vi "Explore Finite Precision Effects.vi"() -> ()   [LabVIEW 2023]
doc: "This example demonstrates the finite word length effects of fixed-point conversion by comparing the error signals of two fixed-point LMS adaptive filters. Each adaptive filter is identical except for the coefficients word length. The first filter has a coefficients word length of 24 bits, and the second filter has a coefficients word length of 16 bits.\n\nAfter you run this VI, this example displays the error signals of both filters. Notice that the error signal of the first filter is smaller than the error signal of the second filter. This difference shows how increasing the coefficients word length reduces errors during fixed-point processing. However, increasing the coefficients word length also increases the amount of hardware resources a filter requires.\n\nOn the block diagram of this example VI, double-click the AFT Simulate Fixed-Point FIR LMS Express VI to examine the settings of the fixed-point LMS adaptive filters. You also can modify the settings to find out how different settings affect the performance of the fixed-point adaptive filters."
uses:
  <vilib>/addons/Adaptive Filters/Utilities/AFT Fixed-Point Settings.ctl
  <vilib>/addons/Adaptive Filters/Utilities/AFT Algorithm.ctl
  <vilib>/addons/Adaptive Filters/Fixed-Point Simulation/LMS/AFT Simulate Fixed-Point FIR LMS.xnode
  <vilib>/addons/Adaptive Filters/NI_AdaptiveFilter.lvlib
  <vilib>/addons/Adaptive Filters/Utilities/AFT Simulation Info.ctl
panel:
  in  "Samples":i32=4096 min=100
  out "Error Signals":dbl[][](graph)
  # "Select Help>>Show Context Help and move the cursor over the VI icon of this example for more information."
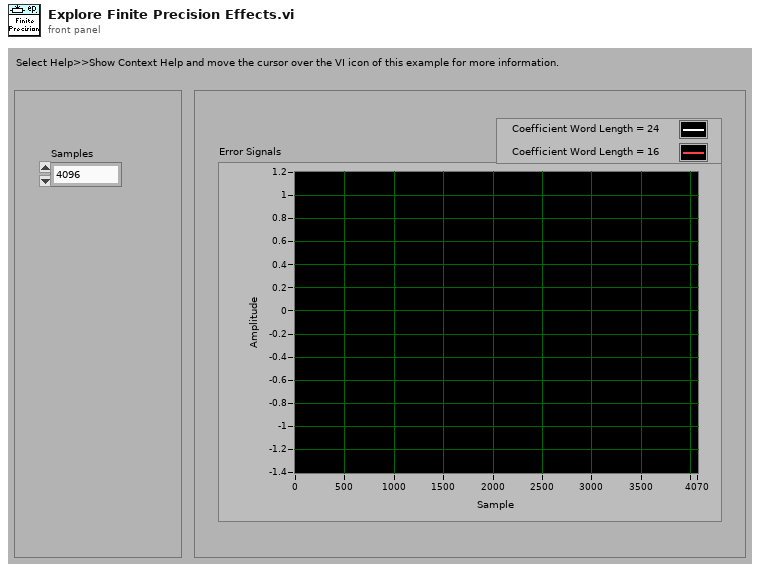
[diagram p1: front panel]
types:
  T1 = typedef "NI_AdaptiveFilter.lvlib/AFT Fixed-Point Settings.ctl" = cluster{"algorithm":u16, "filter length":i32, "step size":dbl, "encoding":cluster{"x(n) word length":i32, "x(n) integer word length":i32, "d(n) word length":i32, "d(n) integer word length":i32, "w(n) word length":i32, "w(n) integer word length":i32, "step size word length":i32, "step size integer word length":i32}}
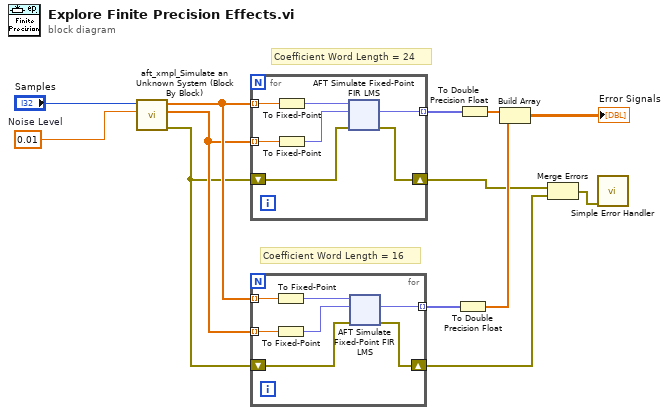
[diagram p0: block diagram]
diagram:
  w4 = 0.01  # Noise Level
  # "Coefficient Word Length = 16"
  # "Coefficient Word Length = 24"
  n1 = call "aft_xmpl_Simulate an Unknown System (Block By Block).vi"("noise level"=w4, "samples"="Samples") -> ("error out"=w1:errorcluster, "response signal"=w2:dbl[], "stimulus signal"=w3:dbl[])  [unwired: 2 in, 5 out]
  n2 = for {
    tunnel: w3 -> [w20] mode=indexing
    tunnel: w2 -> [w18] mode=indexing
    tunnel: [w16] -> w10 mode=indexing
    shift-right: [w15] -> w8
    shift-left: w1 -> [w14]
    n3 = To Fixed-Point(number=w20) -> (fixed-point=w19:fxp<+/-,24,4>)  [unwired: 1 out]
    n4 = To Fixed-Point(number=w18) -> (fixed-point=w17:fxp<+/-,24,4>)  [unwired: 1 out]
    n5 = xnode "AFT Simulate Fixed-Point FIR LMS"("x(n)"=w19, "d(n)"=w17, "error in (no error)"=w14) -> ("e(n)"=w16:fxp<+/-,24,4>, "error out"=w15:errorcluster)  [unwired: 2 in, 4 out]
  }
  n6 = for {
    tunnel: w3 -> [w140] mode=indexing
    tunnel: w2 -> [w138] mode=indexing
    tunnel: [w136] -> w9 mode=indexing
    shift-right: [w135] -> w7
    shift-left: w1 -> [w134]
    n7 = To Fixed-Point(number=w140) -> (fixed-point=w139:fxp<+/-,24,4>)  [unwired: 1 out]
    n8 = To Fixed-Point(number=w138) -> (fixed-point=w137:fxp<+/-,24,4>)  [unwired: 1 out]
    n9 = xnode "AFT Simulate Fixed-Point FIR LMS"("x(n)"=w139, "d(n)"=w137, "error in (no error)"=w134) -> ("e(n)"=w136:fxp<+/-,24,4>, "error out"=w135:errorcluster)  [unwired: 2 in, 4 out]
  }
  n10 = To Double Precision Float(number=w9) -> (double precision float=w13:dbl[])
  n11 = To Double Precision Float(number=w10) -> (double precision float=w12:dbl[])
  n12 = Build Array(w12, w13) -> (→"Error Signals":dbl[][])
  n13 = Merge Errors(w8, w7) -> (w6:errorcluster)
  n14 = call <vilib>:"Simple Error Handler.vi"("error in (no error)"=w6) -> ()  [unwired: 1 in, 8 out]
